vi "send_mark_10_config.vi"(6 "Number of Cycles":i32, 7 "VISA Refnum in":refnum<visa-resource-name>, 8 "error in (no error)":errorcluster, 9 "Down Limit(mm)":dbl, 10 "Up Limit(mm)":dbl, 11 "Speed (mm/min)":dbl) -> (0 "error out":errorcluster, 3 "VISA Refnum out":refnum<visa-resource-name>)   [LabVIEW 2017]
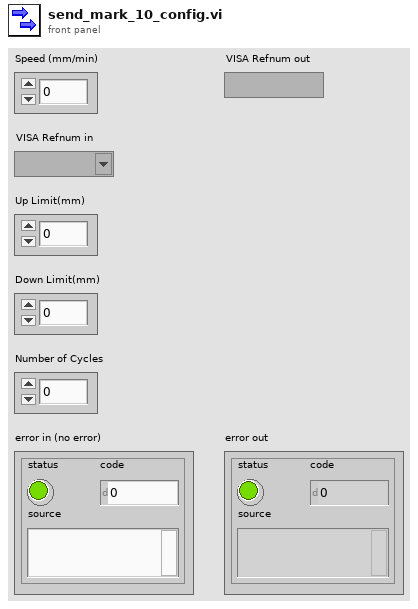
[diagram p1: front panel]
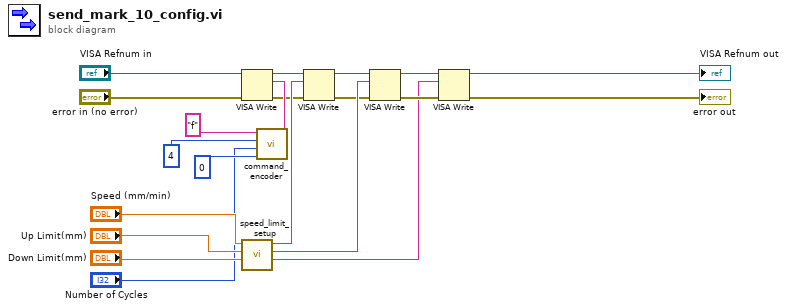
[diagram p0: block diagram]
diagram:
  n1 = call "speed_limit_setup.vi"("Down Limit"="Down Limit(mm)", "Up Limit"="Up Limit(mm)", "Speed"="Speed (mm/min)") -> ("String out"=w1:string, "String out 2"=w6:string, "String out 3"=w9:string)  [unwired: 6 in]
  n2 = call "command_encoder.vi"("String in"="f", "Numeric"=4, "Speed"="Number of Cycles", "Numeric 2"=0) -> ("String out"=w10:string)  [unwired: 6 in]
  n3 = VISA Write(VISA resource name="VISA Refnum in", write buffer=w10, error in (no error)="error in (no error)") -> (VISA resource name out=w8:refnum<visa-resource-name>, error out=w7:errorcluster)  [unwired: 1 out]
  n4 = VISA Write(VISA resource name=w8, write buffer=w9, error in (no error)=w7) -> (VISA resource name out=w4:refnum<visa-resource-name>, error out=w5:errorcluster)  [unwired: 1 out]
  n5 = VISA Write(VISA resource name=w4, write buffer=w6, error in (no error)=w5) -> (VISA resource name out=w3:refnum<visa-resource-name>, error out=w2:errorcluster)  [unwired: 1 out]
  n6 = VISA Write(VISA resource name=w3, write buffer=w1, error in (no error)=w2) -> (VISA resource name out=→"VISA Refnum out":refnum<visa-resource-name>, error out=→"error out":errorcluster)  [unwired: 1 out]
